vi "MAIN_cooler.vi"(3 "error in":errorcluster, 4 "Cooler":bool, 5 "queue CAMERA":refnum<queue>) -> (0 "error out":errorcluster)   [LabVIEW 2015]
uses:
  CONTROLS/Q_camera_element.ctl
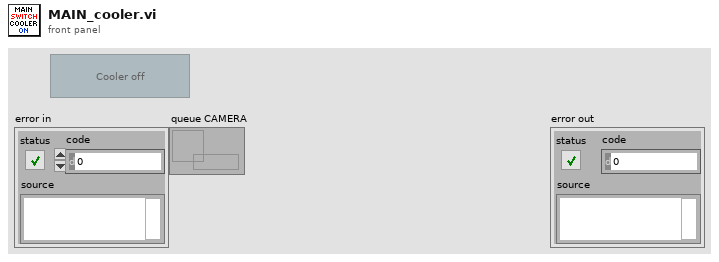
[diagram p1: front panel]
types:
  T1 = typedef "Q_camera_element.ctl" = cluster{"variant":variant, "Instruction":enum16{"CAMERA_idle", "CAMERA_initialize", "CAMERA_error", "CAMERA_security_stop", "CAMERA_not_acquiring", "CAMERA_acquiring", "CAMERA_start_acquiring", "CAMERA_stop_acquiring", "CAMERA_change_exposure", "CAMERA_define_ROI", "CAMERA_cooler", "CAMERA_acquire_movie", "CAMERA_init_scan", "CAMERA_check_new_scan_image", "CAMERA_close_scan", "CAMERA_init_merFISH", "CAMERA_start_acquiring_merFISH", "CAMERA_close_scan_merFISH", "CAMERA_close_merFISH", "CAMERA_STOP"}}
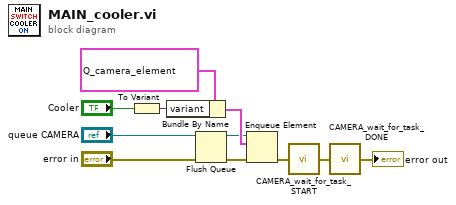
[diagram p0: block diagram]
diagram:
  n1 = To Variant(anything="Cooler") -> (Variant=w4:variant)
  n2 = Bundle By Name(cluster=T1 {"variant"=variant, "Instruction"=enum."CAMERA_cooler"} ("Q_ANDOR_element"), "variant"=w4) -> (w8:T1)
  n3 = Flush Queue(queue="queue CAMERA", error in (no error)="error in") -> (queue out=w7:refnum<queue>, error out=w6:errorcluster)  [unwired: 1 out]
  n4 = Enqueue Element(queue=w7, element=w8, error in (no error)=w6) -> (error out=w10:errorcluster)  [unwired: 1 in, 2 out]
  n5 = call "CAMERA_wait_for_task_START.vi"("error in"=w10) -> ("error out"=w9:errorcluster)
  n6 = call "CAMERA_wait_for_task_DONE.vi"("error in"=w9) -> ("error out"=→"error out":errorcluster)
